vi "send diagnostic info.vi"(7 "Type (Event)":T1(ring), 8 "error in":errorcluster, 10 "Info":string, 11 "node ref":T2) -> (0 "error out":errorcluster, 3 "node ref":T2)   [LabVIEW 2020, in "Publisher Subscriber.lvlib"]
uses:
  Publisher Subscriber.lvlib
  Controls/event info.ctl
  Controls/data cluster.ctl
  Controls/subscription bank ref.ctl
  Controls/node dvr data.ctl
  Controls/node refnum.ctl
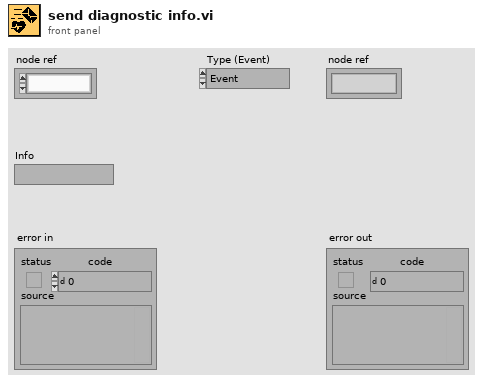
[diagram p1: front panel]
types:
  T1 = enum16{"Event", "Info", "Debug", "Warning", "Error"}
  T2 = typedef "Publisher Subscriber.lvlib/node refnum.ctl" = refnum<k1>
  T3 = typedef "Publisher Subscriber.lvlib/event info.ctl" = cluster{"Module Name":string, "Type":enum16{"Event", "Info", "Debug", "Warning", "Error"}, "Info":string}
  T4 = typedef "Publisher Subscriber.lvlib/node dvr data.ctl" = cluster{"queue ref":refnum<queue>, "Subscription Bank Ref":refnum<data-value>, "Command":string, "Data":variant, "Subscriptions []":set{string}, "Variables DVR Ref":refnum<data-value>, "node name":string}
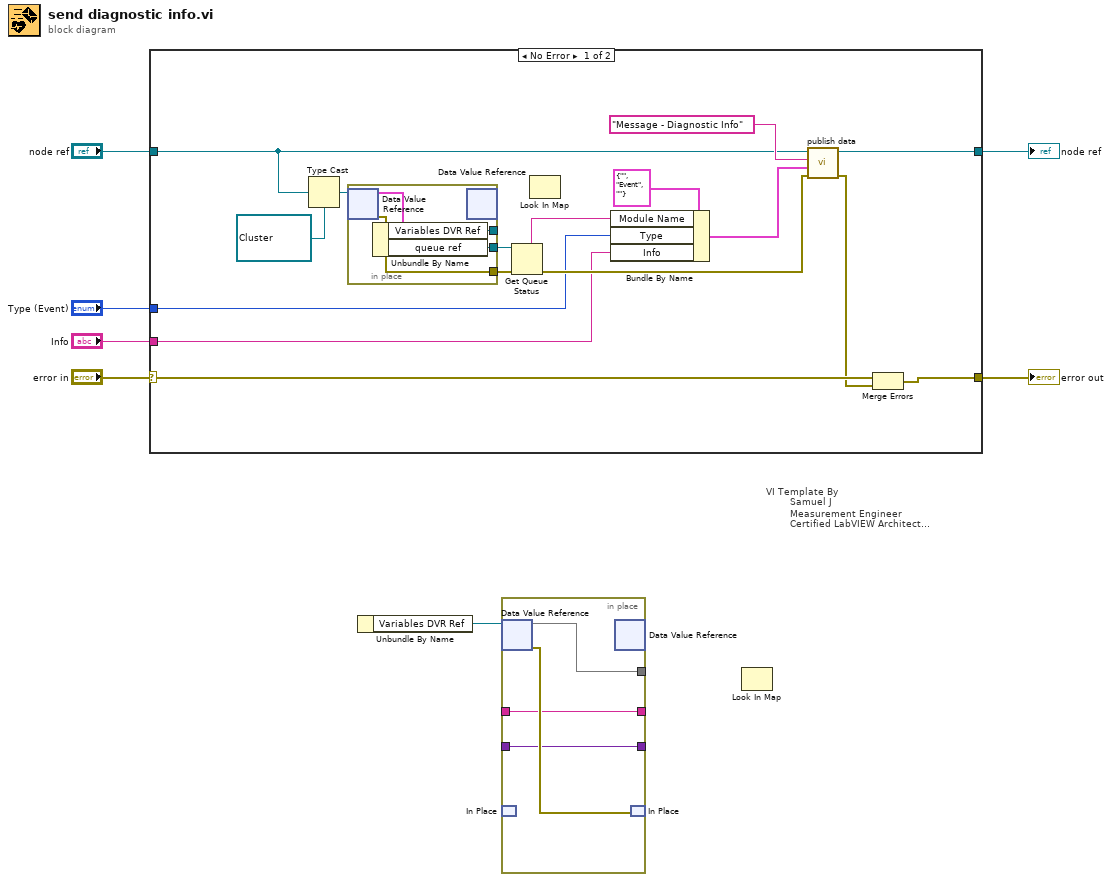
[diagram p0: block diagram]
diagram:
  n1 = case "VI Template By\n        Samuel J\n        Measurement Engineer\n        Certified LabVIEW Architect\n        Vestas Technology R&D Chennai" shown="No Error" "error in" {
    selector: "error in" -> [w28 w38]
    tunnel: [w21 w38] -> w15
    tunnel: "node ref" -> [w26 w37]
    tunnel: [w32 w37] -> w13
    tunnel: "Type (Event)" -> [w18 _]
    tunnel: "Info" -> [w17 _]
    frame No Error {
      n2 = Type Cast(type=refnum<data-value> refnum ("data value reference"), x=w26) -> (*(type *) &x=w25:refnum<data-value>)
      n3 = in-place {
        in-place-border: [w35] -> w24
        in-place-border: [w34] -> w19
        in-place-border: [w33] -> _
        n4 = in-place-dvr #1(w25) -> (w36:T4, w34:errorcluster)
        n5 = Unbundle By Name(w36) -> ("Variables DVR Ref"=w33:refnum<data-value>, "queue ref"=w35:refnum<queue>)
        n6 = in-place-dvr #1() -> ()  [unwired: 1 in, 2 out]
      }
      n7 = Get Queue Status(queue=w24, error in (no error)=w19) -> (queue name=w23:string, error out=w22:errorcluster)  [unwired: 1 in, 6 out]
      n8 = Look In Map() -> ()  [unwired: 3 in, 2 out]
      n9 = Bundle By Name(cluster=T3 {"Module Name"="", "Type"=enum."Event", "Info"=""} ("error info"), "Module Name"=w23, "Type"=w18, "Info"=w17) -> (w30:T3)
      n10 = call "publish data.vi"("error in"=w22, "data in"=w30, "command"="Message - Diagnostic Info", "refnum in"=w26) -> ("error out"=w20:errorcluster, "refnum in"=w32:T2)  [unwired: 6 in]
      n11 = Merge Errors(w28, w20) -> (w21:errorcluster)
    }
    frame Error {
    }
  }
  "error out" <- w15
  "node ref" <- w13
  n12 = Unbundle By Name() -> ("Variables DVR Ref"=w8:refnum<data-value>)  [unwired: 1 in]
  n13 = in-place {
    in-place-border: [w39] -> w7
    in-place-border: [w39] -> w4
    in-place-border: [w40] -> w3
    in-place-border: [w41] -> w2
    in-place-border: [w40] -> w1
    n14 = in-place-dvr #2(w8) -> (w41:map{string, variant}, w42:errorcluster)
    n15 = in-place-match #3() -> (w6:errorcluster)  [unwired: 1 out]
    n16 = in-place-dvr #2() -> ()  [unwired: 1 in, 2 out]
    n17 = in-place-match #3(w42) -> (w5:errorcluster)
  }
  n18 = Look In Map() -> (map=w10:map{string, i32}, key=w9:string)  [unwired: 1 in, 2 out]
